vi "FL Hermite Polynomial COA Single Side.vi"(0 "weight":dbl, 1 "element":T1 {"coa_x(y) coeff" format="%.4g"; "Area(y) coeff" format="%.4g"; "X(y) coeff" format="%.4g"; "Y(x) coeff" format="%.4g"; "Y" format="%.4g"; "X" format="%.4g"}) -> (4 "xlh":dbl format="%#_10f", 6 "area":dbl format="%#_10f", 8 "coa_x":dbl format="%#_10f", 10 "x_l":dbl format="%#_10f", 15 "x_r":dbl format="%#_10f")   [LabVIEW 2017, in "NI_Fuzzy_Logic_API.lvlib"]
uses:
  <vilib>/addons/Fuzzy Logic/NI_Fuzzy_Logic_API.lvlib
  <vilib>/addons/Fuzzy Logic/TypeDefs/FL Interpolating polynomials.ctl
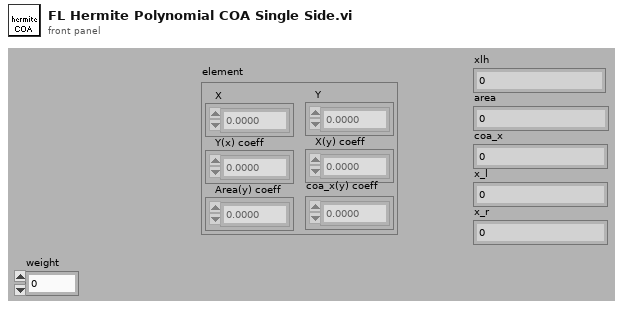
[diagram p1: front panel]
types:
  T1 = typedef "NI_Fuzzy_Logic_API.lvlib/FL Interpolating polynomials.ctl" = cluster{"X":dbl[], "Y":dbl[], "Y(x) coeff":dbl[][], "X(y) coeff":dbl[][], "Area(y) coeff":dbl[][], "coa_x(y) coeff":dbl[][]}
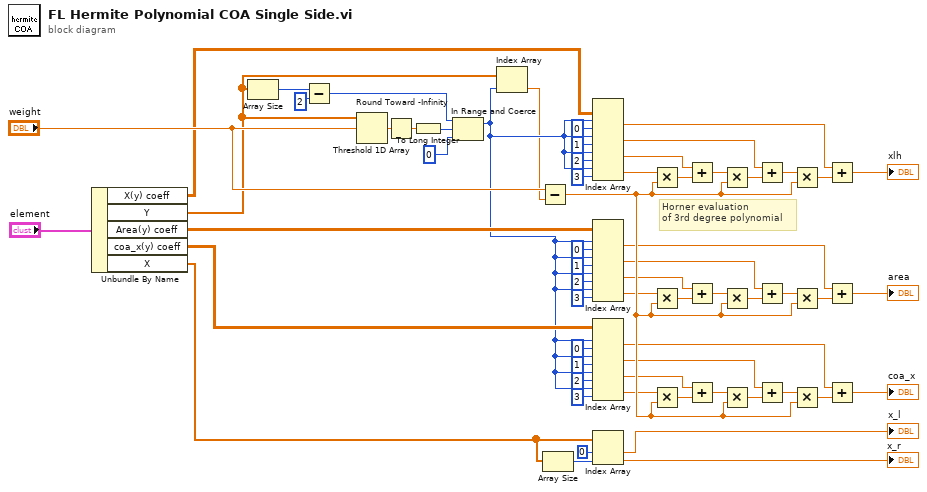
[diagram p0: block diagram]
diagram:
  # "Horner evaluation\nof 3rd degree polynomial"
  n1 = Unbundle By Name("element") -> ("X(y) coeff"=w2:dbl[][], "Y"=w1:dbl[], "Area(y) coeff"=w56:dbl[][], "coa_x(y) coeff"=w57:dbl[][], "X"=w3:dbl[])
  n2 = Array Size(array=w1) -> (size(s)=w26:i32)
  n3 = Subtract(x=w26, y=2) -> (x-y=w27:i32)
  n4 = Threshold 1D Array(2:"weight", 3:w1) -> (0:w23:dbl)  [unwired: 1 out]
  n5 = Round Toward -Infinity(1:w23) -> (0:w22:dbl)
  n6 = To Long Integer(number=w22) -> (32bit integer=w21:i32)
  n7 = In Range and Coerce(upper limit=w27, x=w21, lower limit=0) -> (coerced(x)=w54:i32)  [unwired: 1 out]
  n8 = Index Array(array=w1, index=w54) -> (element=w24:dbl)
  n9 = Subtract(x="weight", y=w24) -> (x-y=w55:dbl)
  n10 = Array Size(array=w3) -> (size(s)=w6:i32)
  n11 = Index Array(array=w2, index (row) #1=w54, index (col) #1=0 ("disabled index (col)"), index (row) #2=w54, index (col) #2=1 ("disabled index (col)"), index (row) #3=w54, index (col) #3=2 ("disabled index (col)"), index (row) #4=w54, index (col) #4=3 ("disabled index (col)")) -> (element #1=w7:dbl, element #2=w10:dbl, element #3=w13:dbl, element #4=w15:dbl)
  n12 = Index Array(array=w56, index (row) #1=w54, index (col) #1=0 ("disabled index (col)"), index (row) #2=w54, index (col) #2=1 ("disabled index (col)"), index (row) #3=w54, index (col) #3=2 ("disabled index (col)"), index (row) #4=w54, index (col) #4=3 ("disabled index (col)")) -> (element #1=w40:dbl, element #2=w37:dbl, element #3=w34:dbl, element #4=w32:dbl)
  n13 = Index Array(array=w57, index (row) #1=w54, index (col) #1=0 ("disabled index (col)"), index (row) #2=w54, index (col) #2=1 ("disabled index (col)"), index (row) #3=w54, index (col) #3=2 ("disabled index (col)"), index (row) #4=w54, index (col) #4=3 ("disabled index (col)")) -> (element #1=w41:dbl, element #2=w44:dbl, element #3=w47:dbl, element #4=w49:dbl)
  n14 = Index Array(array=w3, index #1=0 ("index"), index #2=w6) -> (element #1=→"x_l":dbl, element #2=→"x_r":dbl)
  n15 = Multiply(x=w15, y=w55) -> (x*y=w14:dbl)
  n16 = Multiply(x=w32, y=w55) -> (x*y=w33:dbl)
  n17 = Multiply(x=w49, y=w55) -> (x*y=w48:dbl)
  n18 = Add(x=w13, y=w14) -> (x+y=w12:dbl)
  n19 = Add(x=w34, y=w33) -> (x+y=w35:dbl)
  n20 = Add(x=w47, y=w48) -> (x+y=w46:dbl)
  n21 = Multiply(x=w12, y=w55) -> (x*y=w11:dbl)
  n22 = Multiply(x=w35, y=w55) -> (x*y=w36:dbl)
  n23 = Multiply(x=w46, y=w55) -> (x*y=w45:dbl)
  n24 = Add(x=w10, y=w11) -> (x+y=w9:dbl)
  n25 = Add(x=w37, y=w36) -> (x+y=w38:dbl)
  n26 = Add(x=w44, y=w45) -> (x+y=w43:dbl)
  n27 = Multiply(x=w9, y=w55) -> (x*y=w8:dbl)
  n28 = Multiply(x=w38, y=w55) -> (x*y=w39:dbl)
  n29 = Multiply(x=w43, y=w55) -> (x*y=w42:dbl)
  n30 = Add(x=w7, y=w8) -> (x+y=→"xlh":dbl)
  n31 = Add(x=w40, y=w39) -> (x+y=→"area":dbl)
  n32 = Add(x=w41, y=w42) -> (x+y=→"coa_x":dbl)
